vi "结果判定.vi"(0 "实时数据":string[](array[string])=["1", "0.4"], 1 "限位设定":string[](array[string])=["0.5", "0.1", "0.8", "0.2"], 2 "BarcodeArray":string[](array[string])=["DLXG7007DRWM"], 3 "TimeStartEnd":string[](array[string]), 4 "TestName":string[](array[string]), 5 "MeasurementUnit":string[](array[string]), 6 "Reserved":string="Reserved", 7 "SW_Version":string="1.57") -> (11 "结果字符串":string, 12 "PDCA Data Out":string, 13 "结果状态数组":string[](array[string]), 14 "结果判定":bool[](array[boolean]), 15 "color":u32[](array[numeric]), 16 "结果字符串":string, 17 "结果数组":string[](array[string]), 18 "position":T1[](array[typedef]), 19 "最后判定结果":bool)   [LabVIEW 2011]
uses:
  <vilib>/Utility/miscctls.llb/LVRowAndColumnTypeDef.ctl
panel:
  out "SerialNumber":string
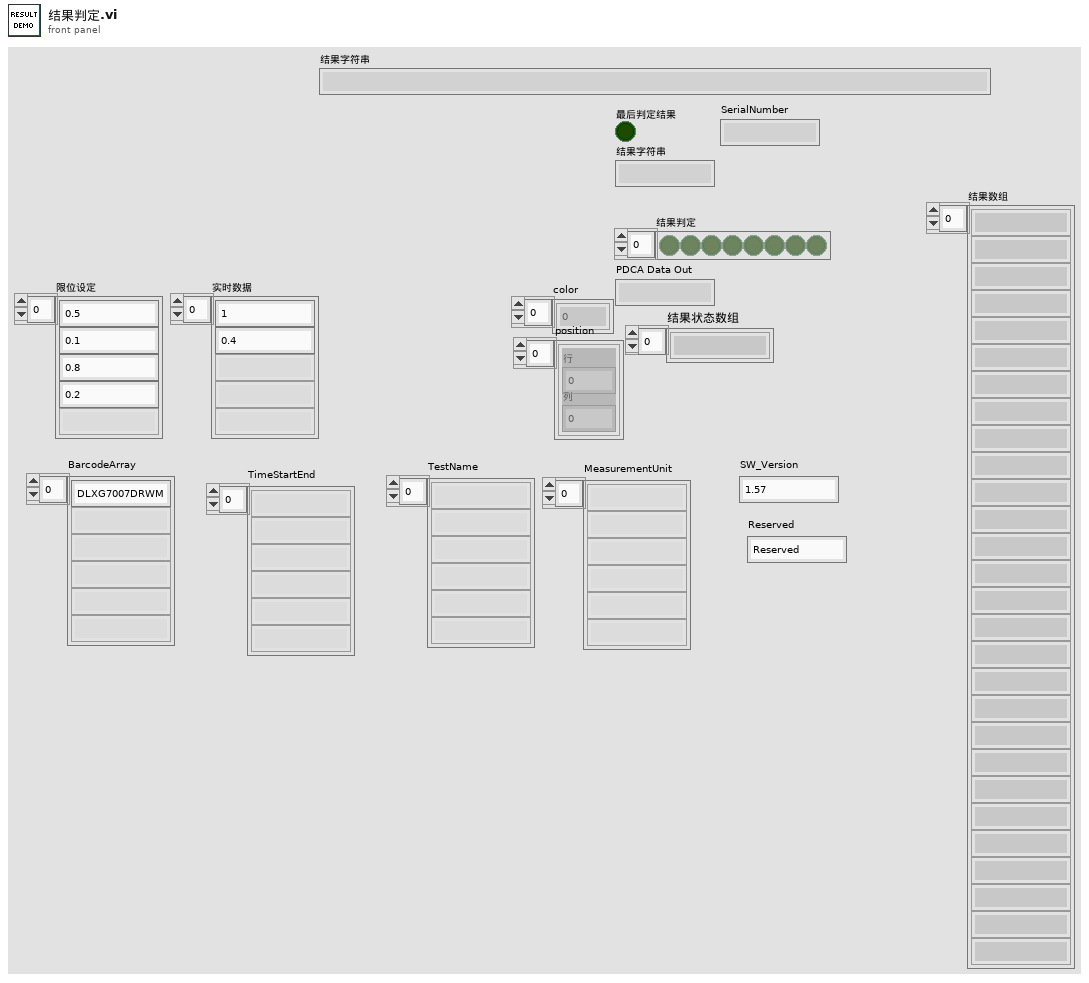
[diagram p1: front panel]
types:
  T1 = typedef "LVRowAndColumnTypeDef.ctl" = cluster{"Row":i32, "Column":i32}
  T2 = cluster{"BarcodeArray":string[], "Limit Array":string[], "Data Array":string[], "TestName Array":string[], "MeasurementUnit Array":string[], "Time Array":string[], "Other Param Array":string[]}
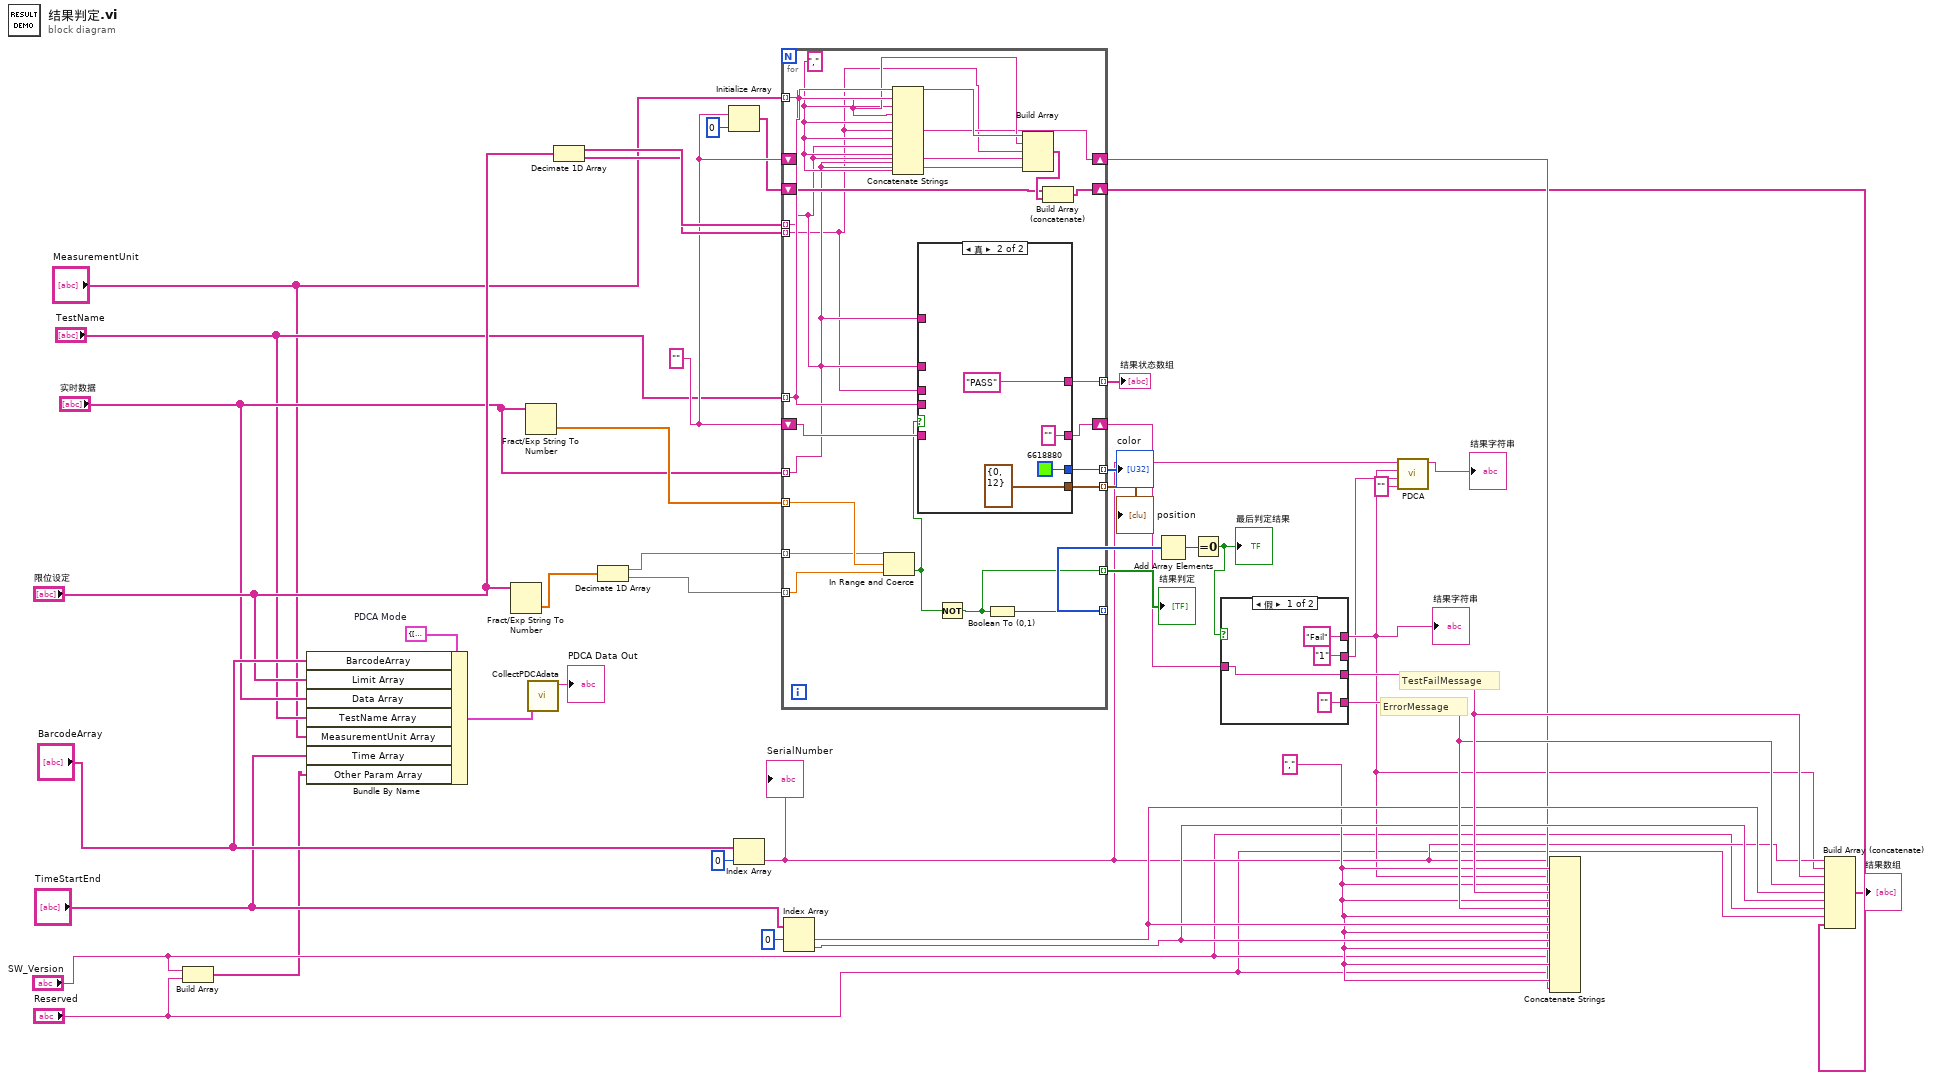
[diagram p0: block diagram]
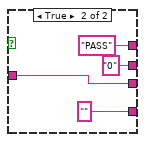
[diagram p2: hidden frame]
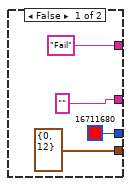
[diagram p3: hidden frame]
diagram:
  w11 = T2 {"BarcodeArray"=[], "Limit Array"=[], "Data Array"=[], "TestName Array"=[], "MeasurementUnit Array"=[], "Time Array"=[], "Other Param Array"=[]}  # PDCA Mode
  w26 = ""
  w29 = ","
  # "ErrorMessage"
  # "TestFailMessage"
  n1 = Build Array("SW_Version", "Reserved") -> (w4:string[])
  n2 = Bundle By Name(cluster=w11, "BarcodeArray"="BarcodeArray", "Limit Array"="限位设定", "Data Array"="实时数据", "TestName Array"="TestName", "MeasurementUnit Array"="MeasurementUnit", "Time Array"="TimeStartEnd", "Other Param Array"=w4) -> (w3:T2)
  n3 = Fract/Exp String To Number(string="限位设定") -> (number=w44:dbl[])  [unwired: 3 in, 1 out]
  n4 = Fract/Exp String To Number(string="实时数据") -> (number=w43:dbl[])  [unwired: 3 in, 1 out]
  n5 = call "CollectPDCAdata.vi"("PDCA Collect Data In"=w3) -> ("PDCA Data Out"=→"PDCA Data Out":string)  [unwired: 10 in]
  n6 = Decimate 1D Array("限位设定") -> (w28:string[], w27:string[])
  n7 = Decimate 1D Array(w44) -> (w42:dbl[], w41:dbl[])
  n8 = Initialize Array(w26, 0 ("维数大小")) -> (w24:string[])
  n9 = Index Array(array="BarcodeArray", index=0 ("索引")) -> (element=w18:string)
  "SerialNumber" <- w18
  n10 = for {
    tunnel: w43 -> [w66] mode=indexing
    tunnel: w42 -> [w65] mode=indexing
    tunnel: w41 -> [w64] mode=indexing
    tunnel: [w49] -> w40 mode=indexing
    tunnel: [w63] -> w39 mode=indexing
    tunnel: "TestName" -> [w60] mode=indexing
    shift-right: [w61] -> w33
    shift-left: w26 -> [w62]
    tunnel: "MeasurementUnit" -> [w59] mode=indexing
    tunnel: w28 -> [w47] mode=indexing
    tunnel: w27 -> [w46] mode=indexing
    tunnel: "实时数据" -> [w48] mode=indexing
    shift-right: [w56] -> w23
    shift-left: w26 -> [w57]
    shift-right: [w53] -> w22
    shift-left: w24 -> [w54]
    tunnel: [w52] -> w19 mode=indexing
    tunnel: [w51] -> w20 mode=indexing
    tunnel: [w45] -> w1 mode=indexing
    w58 = "," ("字符串")
    n11 = In Range and Coerce(upper limit=w65, x=w66, lower limit=w64) -> (In Range?=w50:bool)  [unwired: 1 out]
    n12 = Concatenate Strings(w57, w60, w58, w59, w58, w46, w58, w47, w58, w48, w58) -> (w56:string)
    n13 = case shown="真" w50 {
      tunnel: w60 -> [_ _]
      tunnel: w62 -> [_ _]
      tunnel: ["" ("字符串") "" ("字符串")] -> w61
      tunnel: [T1 {"Row"=0, "Column"=12} ("活动单元格:活动单元格") T1 {"Row"=0, "Column"=12} ("活动单元格:活动单元格")] -> w52
      tunnel: [u32 16711680 u32 6618880] -> w51
      tunnel: w48 -> [_ _]
      tunnel: w48 -> [_ _]
      tunnel: w47 -> [_ _]
      tunnel: w46 -> [_ _]
      tunnel: ["Fail" "PASS" ("字符串")] -> w45
      frame False {
      }
      frame True {
      }
    }
    n14 = Not(x=w50) -> (.not. x?=w49:bool)
    n15 = Boolean To (0,1)(Boolean=w49) -> (0, 1=w63:i16)
    n16 = Build Array(w60, w59, w46, w47, w48) -> (w55:string[])
    n17 = Build Array (concatenate)(w54, w55) -> (w53:string[])
  }
  "结果判定" <- w40
  "color" <- w20
  "position" <- w19
  "结果状态数组" <- w1
  n18 = Index Array(array="TimeStartEnd", index #1=0 ("索引")) -> (element #1=w31:string, element #2=w30:string)  [unwired: 1 in]
  n19 = Add Array Elements(numeric array=w39) -> (sum=w38:i16)
  n20 = Equal To 0?(x=w38) -> (x = 0?=w37:bool)
  "最后判定结果" <- w37
  n21 = case shown="假" w37 {
    tunnel: ["Fail" "PASS"] -> w17
    tunnel: [w77 w79] -> w35
    tunnel: ["" ""] -> w34
    tunnel: w33 -> [w77 w79]
    tunnel: ["1" "0"] -> w16
    frame False {
    }
    frame True {
    }
  }
  "结果字符串" <- w17
  n22 = call "PDCA.vi"("WorkOrde"="", "Errorcode"=w16, "Result"=w17, "SN"=w18) -> ("LineResult"=→"结果字符串":string)  [unwired: 7 in]
  n23 = Concatenate Strings(w18, w29, w17, w29, w35, w29, w34, w29, w31, w29, w30, w29, "SW_Version", w29, "Reserved", w29, w23) -> ()  [unwired: 1 out]
  n24 = Build Array (concatenate)(w18, w17, w35, w34, w31, w30, "SW_Version", "Reserved", w22) -> (→"结果数组":string[])
